vi "Cleanup Session.vi"(8 "error in":errorcluster, 11 "Plugin in":refnum<class "RPM Plugin.lvclass">) -> (0 "error out":errorcluster, 3 "Plugin out":refnum<class "RPM Plugin.lvclass">)   [LabVIEW 2020, in "RPM Plugin.lvlib" / "RPM Plugin.lvclass"]
uses:
  RPM Plugin.lvclass
  RPM Plugin.lvclass/RPM Plugin.ctl
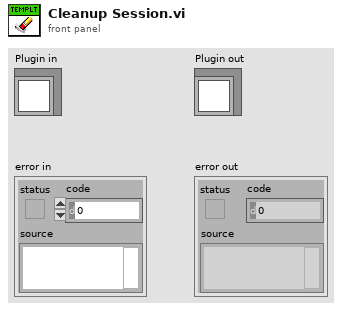
[diagram p1: front panel]
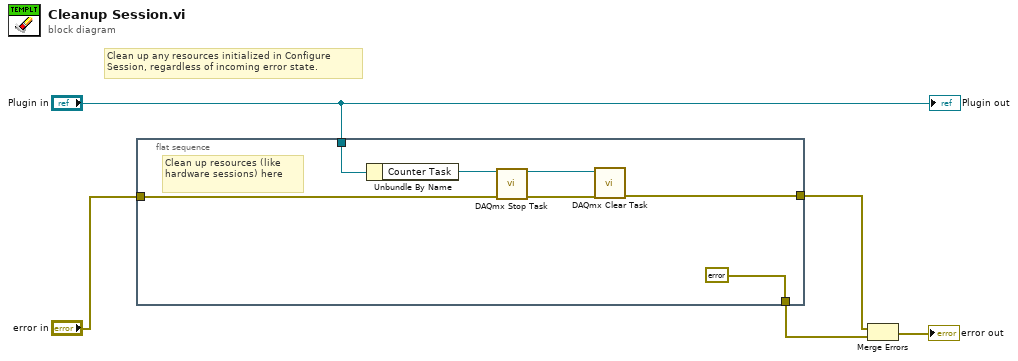
[diagram p0: block diagram]
diagram:
  # "Clean up any resources initialized in Configure Session, regardless of incoming error state."
  n1 = flat-sequence {
    tunnel: [errorcluster {"status"=FALSE, "code"=0, "source"=""} ("error in")] -> w4
    tunnel: "Plugin in" -> [w12]
    tunnel: "error in" -> [w7]
    tunnel: [w6] -> w1
    frame #0 {
      # "Clean up resources (like hardware sessions) here"
      n2 = Unbundle By Name(w12) -> ("Counter Task"=w11:refnum<k21>)
      n3 = call <vilib>:"DAQmx Stop Task.vi"("task/channels in"=w11, "error in"=w7) -> ("task out"=w9:refnum<k21>, "error out"=w8:errorcluster)  [unwired: 12 in]
      n4 = call <vilib>:"DAQmx Clear Task.vi"("task in"=w9, "error in"=w8) -> ("error out"=w6:errorcluster)  [unwired: 13 in]
    }
  }
  n5 = Merge Errors(w1, w4) -> (→"error out":errorcluster)
  "Plugin out" <- "Plugin in"
